vi "Func-Math-Finder.vi"(4 "All Fn-Math":string[](array[string]), 6 "All Fn Name":string[](array[string]), 7 "Func Name":string, 8 "error in (no error)":errorcluster, 11 "Get Tagged String":string) -> (0 "error out":errorcluster, 1 "is empty?":string, 2 "Expression":string)   [LabVIEW 2014]
doc: "This VI takes tagged string from SBML parser.vi as input and translate it into kinetic law. It supports the following five mathematical functions:\n+, -, *, /, pow\n\nDesigned by HB\nhaba@dtu.dk"
uses:
  <vilib>/regexp/Match Regular Expression.xnode
panel:
  out "RHS ex":string
  out "Inter. exp":string
  in  "RHS":string
  in  "LHS":string
  # "SOP1 + x 2 EOP1"
  # "SOP1 + SOP2 * a b EOP2 c EOP1"
  # "SOP1 + c SOP2 * a b EOP2 EOP1"
  # "SOP1 + SOP2 * a SOP3 pow x 2 EOP3 EOP2 SOP2 * b x EOP2 c EOP1"
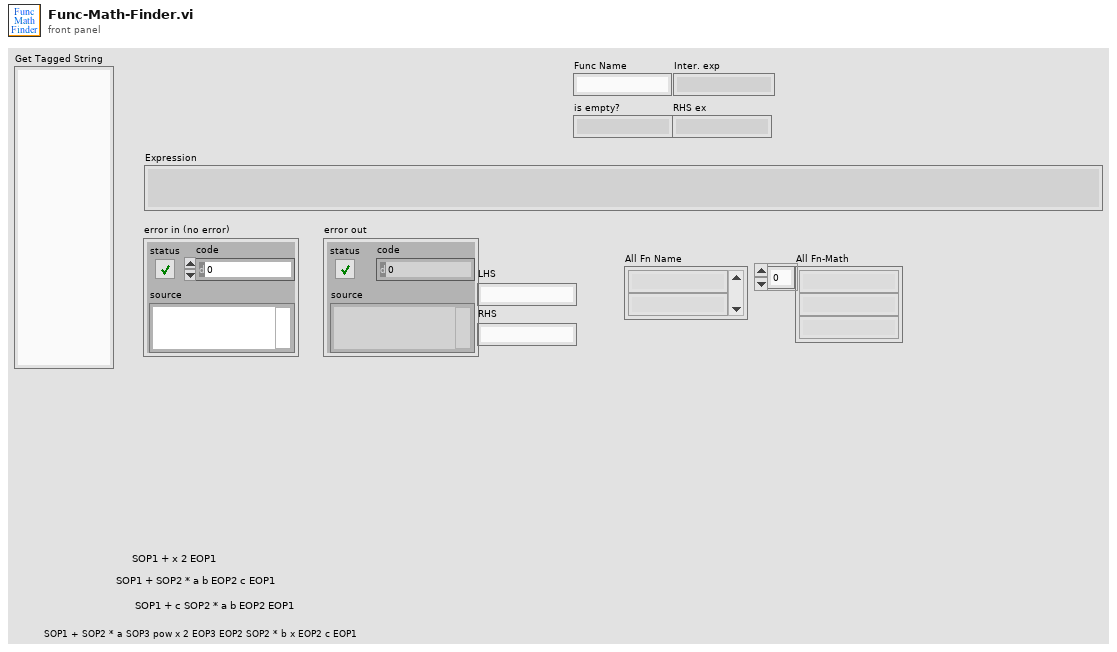
[diagram p1: front panel]
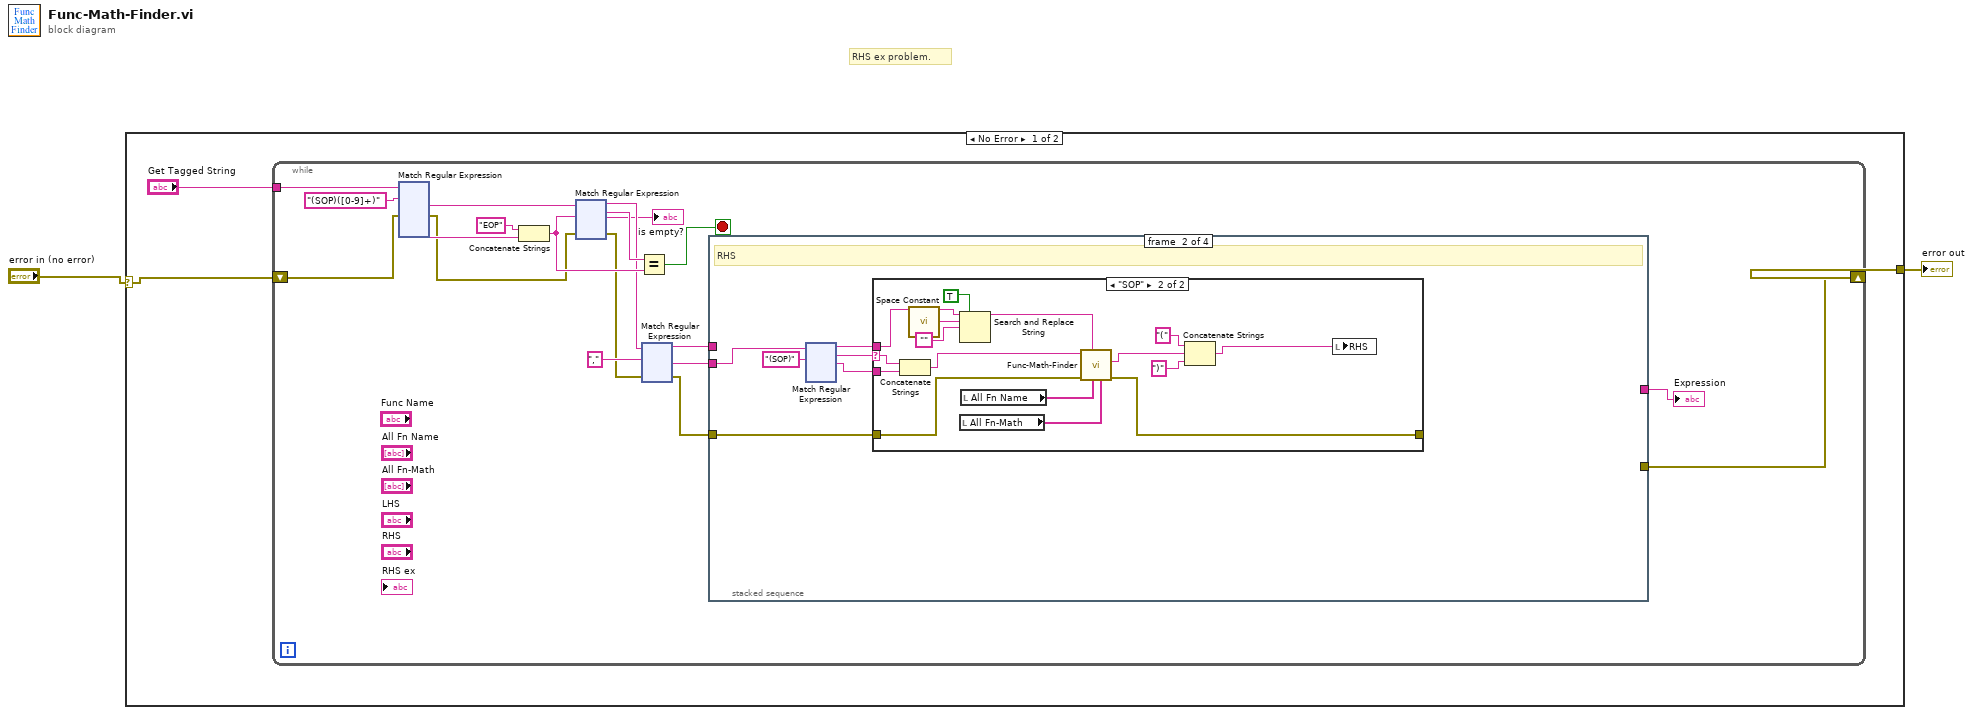
[diagram p0: block diagram]
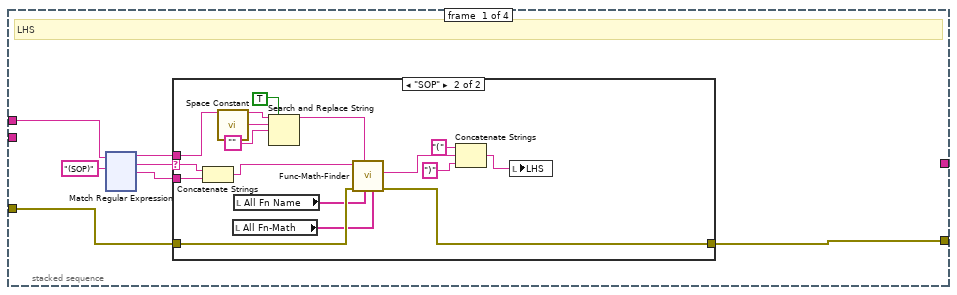
[diagram p2: hidden frame]
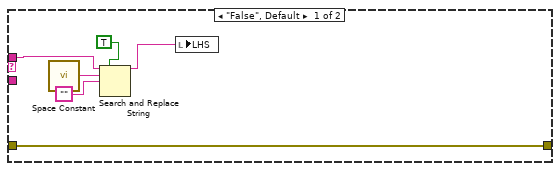
[diagram p3: hidden frame]
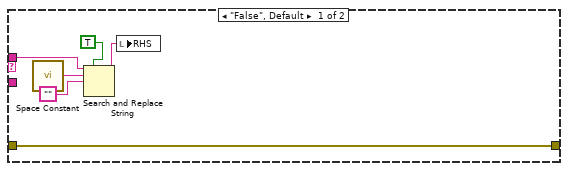
[diagram p4: hidden frame]
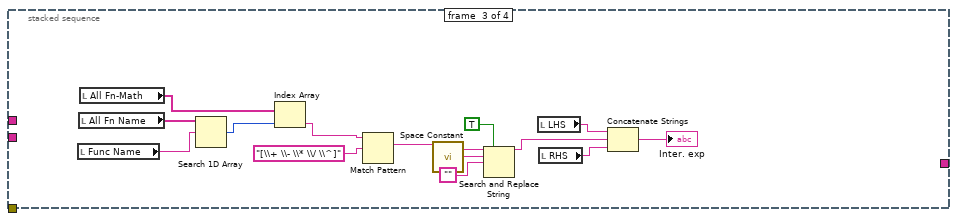
[diagram p5: hidden frame]
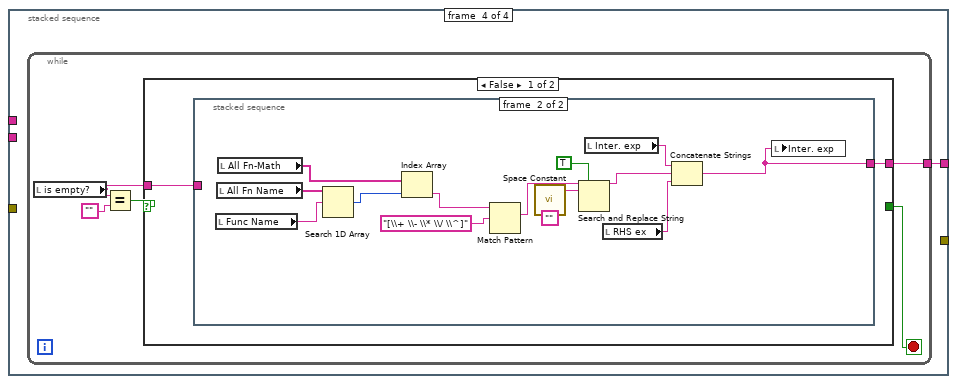
[diagram p6: hidden frame]
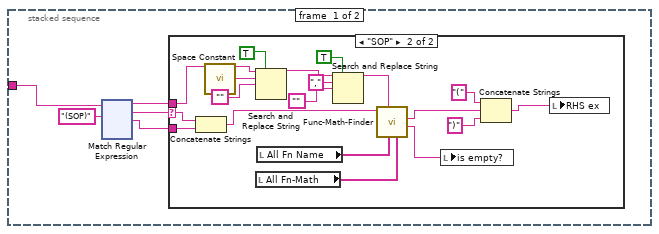
[diagram p7: hidden frame]
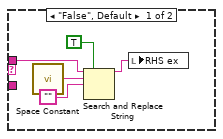
[diagram p8: hidden frame]
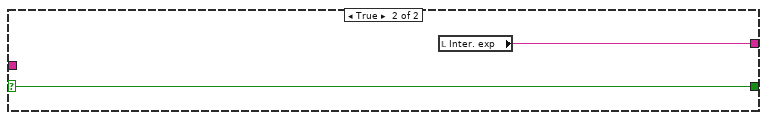
[diagram p9: hidden frame]
diagram:
  # "RHS ex problem."
  n1 = case shown="No Error" "error in (no error)" {
    selector: "error in (no error)" -> [w3 w835]
    tunnel: [w4 w835] -> w2
    frame No Error {
      n2 = while {
        tunnel: "Get Tagged String" -> [w15]
        shift-right: [w10] -> w4
        shift-left: w3 -> [w14]
        stop <- w22 stop-if-true
        n3 = xnode "Match Regular Expression"("input string"=w15, "regular expression"="(SOP)([0-9]+)", "error in"=w14) -> ("after match"=w18:string, "error out"=w13:errorcluster, "submatch 2"=w17:string)  [unwired: 3 in, 4 out]
        n4 = Concatenate Strings("EOP" ("regular expression"), w17) -> (w23:string)
        n5 = xnode "Match Regular Expression"("input string"=w18, "regular expression"=w23, "error in"=w13) -> ("before match"=w20:string, "whole match"=w21:string, "after match"=→"is empty?":string, "error out"=w12:errorcluster)  [unwired: 3 in, 1 out]
        n6 = Equal?(x=w21, y=w23) -> (x = y?=w22:bool)
        n7 = xnode "Match Regular Expression"("input string"=w20, "regular expression"="," ("Oprts Lst"), "error in"=w12) -> ("before match"=w11:string, "after match"=w8:string, "error out"=w9:errorcluster)  [unwired: 3 in, 2 out]
        n8 = stacked-sequence {
          tunnel: w11 -> [w30 _ _ _]
          tunnel: [w27 _ _ _] -> w10
          tunnel: w9 -> [w26 w171 _ _]
          tunnel: w8 -> [_ w170 _ _]
          tunnel: [_ _ _ w324] -> w7
          frame #0 {
            # "LHS"
            n9 = xnode "Match Regular Expression"("input string"=w30, "regular expression"="(SOP)") -> ("before match"=w28:string, "whole match"=w29:string, "after match"=w25:string)  [unwired: 4 in, 2 out]
            n10 = case shown="\"SOP\"" w29 {
              selector: w29 -> [_ w47]
              tunnel: w28 -> [w33 w42]
              tunnel: [w37 w53] -> w27
              tunnel: w26 -> [w37 w52]
              tunnel: w25 -> [_ w46]
              frame "False", Default {
                n11 = call <vilib>:"Space Constant.vi"() -> ("String"=w35:string)
                n12 = Search and Replace String(replace all?=TRUE ("replace all? (F)"), input string=w33, search string=w35, replace string="" ("string")) -> (result string=w32:string)  [unwired: 4 in, 3 out]
                n13 = local write "LHS"(w32) -> ()
              }
              frame "SOP" {
                n14 = Concatenate Strings(w47, w46) -> (w38:string)
                n15 = call <vilib>:"Space Constant.vi"() -> ("String"=w43:string)
                n16 = local read "All Fn-Math"() -> (w39:string[])
                n17 = local read "All Fn Name"() -> (w40:string[])
                n18 = Search and Replace String(replace all?=TRUE ("replace all? (F)"), input string=w42, search string=w43, replace string="" ("string")) -> (result string=w41:string)  [unwired: 4 in, 3 out]
                n19 = call "Func-Math-Finder.vi"("All Fn-Math"=w39, "All Fn Name"=w40, "Func Name"=w41, "error in (no error)"=w52, "Get Tagged String"=w38) -> ("error out"=w53:errorcluster, "Expression"=w51:string)  [unwired: 4 in, 1 out]
                n20 = Concatenate Strings("(" ("string"), w51, ")" ("string")) -> (w48:string)
                n21 = local write "LHS"(w48) -> ()
              }
            }
          }
          frame #1 {
            # "RHS"
            n22 = xnode "Match Regular Expression"("input string"=w170, "regular expression"="(SOP)") -> ("before match"=w168:string, "whole match"=w172:string, "after match"=w169:string)  [unwired: 4 in, 2 out]
            n23 = case shown="\"SOP\"" w172 {
              selector: w172 -> [_ w193]
              tunnel: w168 -> [w175 w183]
              tunnel: [w179 w195] -> _
              tunnel: w171 -> [w179 w194]
              tunnel: w169 -> [_ w192]
              frame "False", Default {
                n24 = call <vilib>:"Space Constant.vi"() -> ("String"=w177:string)
                n25 = Search and Replace String(replace all?=TRUE ("replace all? (F)"), input string=w175, search string=w177, replace string="" ("string")) -> (result string=w174:string)  [unwired: 4 in, 3 out]
                n26 = local write "RHS"(w174) -> ()
              }
              frame "SOP" {
                n27 = Concatenate Strings(w193, w192) -> (w191:string)
                n28 = call <vilib>:"Space Constant.vi"() -> ("String"=w184:string)
                n29 = Search and Replace String(replace all?=TRUE ("replace all? (F)"), input string=w183, search string=w184, replace string="" ("string")) -> (result string=w182:string)  [unwired: 4 in, 3 out]
                n30 = local read "All Fn-Math"() -> (w180:string[])
                n31 = local read "All Fn Name"() -> (w181:string[])
                n32 = call "Func-Math-Finder.vi"("All Fn-Math"=w180, "All Fn Name"=w181, "Func Name"=w182, "error in (no error)"=w194, "Get Tagged String"=w191) -> ("error out"=w195:errorcluster, "Expression"=w187:string)  [unwired: 4 in, 1 out]
                n33 = Concatenate Strings("(" ("string"), w187, ")" ("string")) -> (w188:string)
                n34 = local write "RHS"(w188) -> ()
              }
            }
          }
          frame #2 {
            n35 = local read "Func Name"() -> (w311:string)
            n36 = local read "All Fn Name"() -> (w313:string[])
            n37 = local read "All Fn-Math"() -> (w312:string[])
            n38 = Search 1D Array(1D array=w313, element=w311) -> (index of element=w315:i32)  [unwired: 1 in]
            n39 = Index Array(array=w312, index=w315) -> (element=w314:string)
            n40 = Match Pattern(string=w314, regular expression="[\\+ \\- \\* \\/ \\^]" ("Oprts Lst")) -> (match substring=w316:string)  [unwired: 1 in, 3 out]
            n41 = call <vilib>:"Space Constant.vi"() -> ("String"=w321:string)
            n42 = Search and Replace String(replace all?=TRUE ("replace all? (F)"), input string=w316, search string=w321, replace string="" ("string")) -> (result string=w323:string)  [unwired: 4 in, 3 out]
            n43 = local read "LHS"() -> (w319:string)
            n44 = local read "RHS"() -> (w318:string)
            n45 = Concatenate Strings(w319, w323, w318) -> (→"Inter. exp":string)
          }
          frame #3 {
            n46 = while {
              tunnel: [w326] -> w324
              stop <- w327 stop-if-true
              n47 = local read "is empty?"() -> (w325:string)
              n48 = Equal?(x=w325, y="") -> (x = y?=w328:bool)
              n49 = case shown="False" w328 {
                selector: w328 -> [_ w489]
                tunnel: [_ w489] -> w327
                tunnel: [w330 w488] -> w326
                tunnel: w325 -> [w331 _]
                frame False {
                  n50 = stacked-sequence {
                    tunnel: w331 -> [w332 _]
                    tunnel: [_ w482] -> w330
                    frame #0 {
                      n51 = xnode "Match Regular Expression"("input string"=w332, "regular expression"="(SOP)") -> ("before match"=w333:string, "whole match"=w335:string, "after match"=w334:string)  [unwired: 4 in, 2 out]
                      n52 = case shown="\"SOP\"" w335 {
                        selector: w335 -> [_ w360]
                        tunnel: w333 -> [w338 w350]
                        tunnel: w334 -> [_ w359]
                        frame "False", Default {
                          n53 = call <vilib>:"Space Constant.vi"() -> ("String"=w340:string)
                          n54 = Search and Replace String(replace all?=TRUE ("replace all? (F)"), input string=w338, search string=w340, replace string="" ("string")) -> (result string=w337:string)  [unwired: 4 in, 3 out]
                          n55 = local write "RHS ex"(w337) -> ()
                        }
                        frame "SOP" {
                          n56 = Concatenate Strings(w360, w359) -> (w358:string)
                          n57 = call <vilib>:"Space Constant.vi"() -> ("String"=w351:string)
                          n58 = Search and Replace String(replace all?=TRUE ("replace all? (F)"), input string=w350, search string=w351, replace string="" ("string")) -> (result string=w345:string)  [unwired: 4 in, 3 out]
                          n59 = local read "All Fn-Math"() -> (w348:string[])
                          n60 = local read "All Fn Name"() -> (w349:string[])
                          n61 = Search and Replace String(replace all?=TRUE ("replace all? (F)"), input string=w345, search string=",", replace string="" ("string")) -> (result string=w343:string)  [unwired: 4 in, 3 out]
                          n62 = call "Func-Math-Finder.vi"("All Fn-Math"=w348, "All Fn Name"=w349, "Func Name"=w343, "Get Tagged String"=w358) -> ("is empty?"=w342:string, "Expression"=w354:string)  [unwired: 5 in, 1 out]
                          n63 = local write "is empty?"(w342) -> ()
                          n64 = Concatenate Strings("(" ("string"), w354, ")" ("string")) -> (w355:string)
                          n65 = local write "RHS ex"(w355) -> ()
                        }
                      }
                    }
                    frame #1 {
                      (unwired) "" ("string")
                      n66 = local read "Func Name"() -> (w476:string)
                      n67 = local read "All Fn Name"() -> (w478:string[])
                      n68 = local read "All Fn-Math"() -> (w477:string[])
                      n69 = Search 1D Array(1D array=w478, element=w476) -> (index of element=w480:i32)  [unwired: 1 in]
                      n70 = Index Array(array=w477, index=w480) -> (element=w479:string)
                      n71 = Match Pattern(string=w479, regular expression="[\\+ \\- \\* \\/ \\^]" ("Oprts Lst")) -> (match substring=w475:string)  [unwired: 1 in, 3 out]
                      n72 = call <vilib>:"Space Constant.vi"() -> ("String"=w486:string)
                      n73 = Search and Replace String(replace all?=TRUE ("replace all? (F)"), input string=w475, search string=w486) -> (result string=w485:string)  [unwired: 5 in, 3 out]
                      n74 = local read "Inter. exp"() -> (w484:string)
                      n75 = local read "RHS ex"() -> (w483:string)
                      n76 = Concatenate Strings(w484, w485, w483) -> (w482:string)
                      n77 = local write "Inter. exp"(w482) -> ()
                    }
                  }
                }
                frame True {
                  n78 = local read "Inter. exp"() -> (w488:string)
                }
              }
            }
          }
        }
        "Expression" <- w7
      }
    }
    frame Error {
    }
  }
  "error out" <- w2
